vi "Sequence Tester.vi"() -> ()   [LabVIEW 2014, in "SimSyA.lvlib"]
uses:
  SimSyA.lvlib
  DriverMasterSync/build/DriverMasterSync.lvlibp/APIs/Data Queue/Acquisition Data Cluster.ctl
  DriverMasterSync/build/DriverMasterSync.lvlibp/APIs/Data Queue/Acquisition Data 1 Sample Cluster.ctl
  DriverMasterSync/build/DriverMasterSync.lvlibp/APIs/Data Queue/Control Data Cluster.ctl
  SimSyAClass/SimSyA.lvclass
  DriverMasterSync/build/DriverMasterSync.lvlibp/APIs/Data Queue/WINFAS 2 Data Queue.lvlib
panel:
  out "Control Data":T1
  out "Acquisition Data":T2
  in  "stop":bool
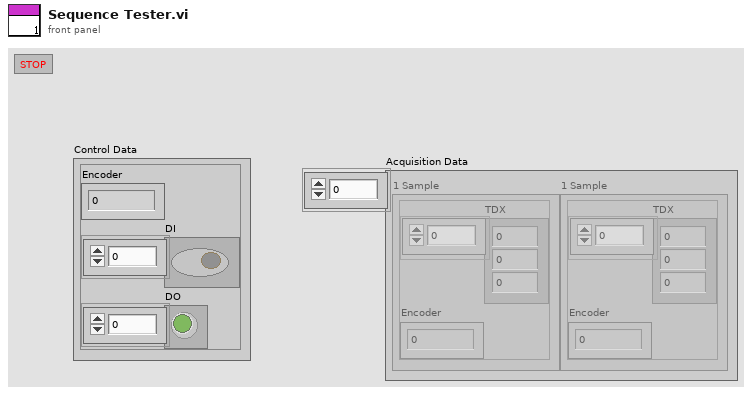
[diagram p1: front panel]
types:
  T1 = typedef "DriverMasterSync.lvlibp/WINFAS 2 Data Queue.lvlib/Control Data Cluster.ctl" = cluster{"Encoder":sgl, "DI":bool[], "DO":bool[]}
  T2 = typedef "DriverMasterSync.lvlibp/WINFAS 2 Data Queue.lvlib/Acquisition Data Cluster.ctl" = T3[]
  T3 = typedef "DriverMasterSync.lvlibp/WINFAS 2 Data Queue.lvlib/Acquisition Data 1 Sample Cluster.ctl" = cluster{"TDX":sgl[], "Encoder":sgl}
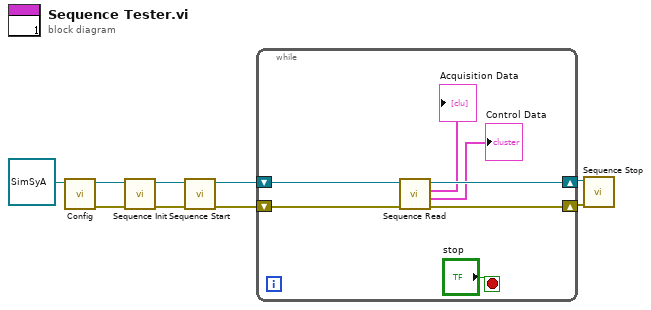
[diagram p0: block diagram]
diagram:
  n1 = call-dynamic "Config.vi"("SimSyA in"=refnum<class "SimSyA.lvclass"> refnum) -> ("error out"=w4:errorcluster, "SimSyA out"=w9:refnum<class "SimSyA.lvclass">)  [unwired: 8 in, 1 out]
  n2 = call-dynamic "Sequence Init.vi"("error in (no error)"=w4, "SimSyA in"=w9) -> ("error out"=w3:errorcluster, "SimSyA out"=w8:refnum<class "SimSyA.lvclass">)  [unwired: 8 in]
  n3 = call-dynamic "Sequence Start.vi"("error in (no error)"=w3, "SimSyA in"=w8) -> ("error out"=w2:errorcluster, "SimSyA out"=w7:refnum<class "SimSyA.lvclass">)  [unwired: 8 in]
  n4 = while {
    shift-right: [w15] -> w6
    shift-left: w7 -> [w16]
    shift-right: [w13] -> w1
    shift-left: w2 -> [w14]
    stop <- "stop" stop-if-true
    n5 = call-dynamic "Sequence Read.vi"("error in (no error)"=w14, "SimSyA in"=w16) -> ("error out"=w13:errorcluster, "Control Data"=→"Control Data":T1, "Acquisition Data"=→"Acquisition Data":T2, "SimSyA out"=w15:refnum<class "SimSyA.lvclass">)  [unwired: 6 in]
  }
  n6 = call-dynamic "Sequence Stop.vi"("error in (no error)"=w1, "SimSyA in"=w6) -> ()  [unwired: 8 in, 2 out]
